vi "DerotatorControl_byYaw.vi"() -> ()   [LabVIEW 2020]
uses:
  <vilib>/DAQmx/write.llb/DAQmx Write (Digital Bool 1Line 1Point).vi
  <vilib>/DAQmx/create/channels.llb/DAQmx Create Channel (DO-Digital Output).vi
  <vilib>/DAQmx/miscellaneous.llb/DAQmx Fill In Error Info.vi
  GlobalYAW.vi
panel:
  in  "step":bool
  in  "stop":bool
  in  "Record!":bool
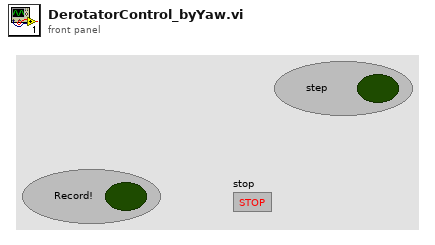
[diagram p1: front panel]
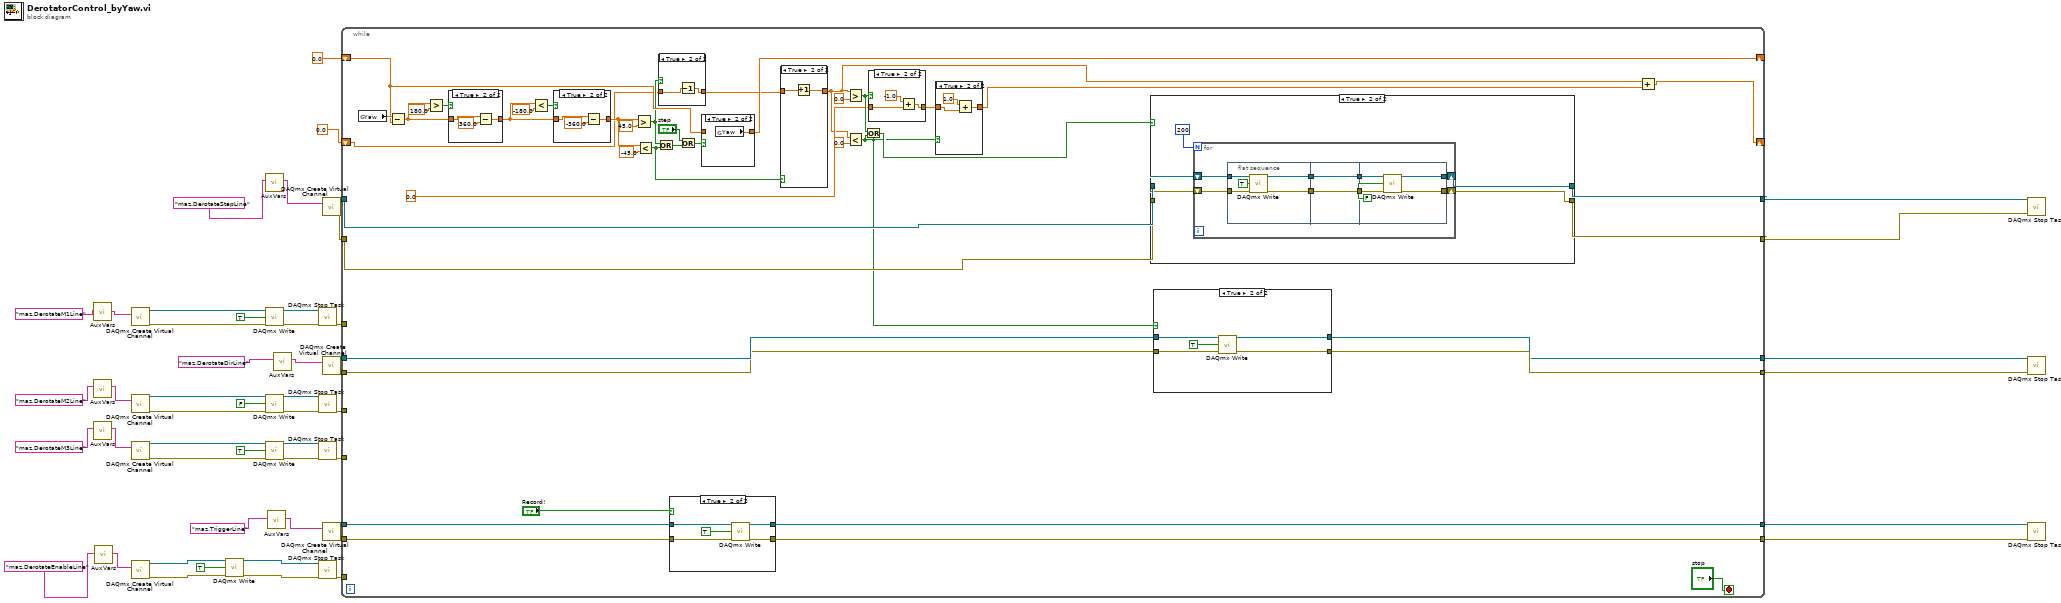
[diagram p0: block diagram]
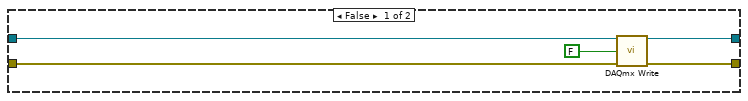
[diagram p9: hidden frame]
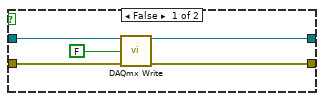
[diagram p10: hidden frame]
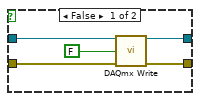
[diagram p11: hidden frame]
diagram:
  n1 = call "AuxVars.vi"("key"="maz.DerotateM1Line") -> ("value"=w15:string)  [unwired: 9 in, 1 out]
  n2 = call "AuxVars.vi"("key"="maz.DerotateM2Line") -> ("value"=w9:string)  [unwired: 9 in, 1 out]
  n3 = call "AuxVars.vi"("key"="maz.DerotateM3Line") -> ("value"=w7:string)  [unwired: 9 in, 1 out]
  n4 = call "AuxVars.vi"("key"="maz.DerotateEnableLine") -> ("value"=w5:string)  [unwired: 9 in, 1 out]
  n5 = call-poly <vilib>:"DAQmx Create Virtual Channel.vi"("lines"=w15) -> ("task out"=w34:refnum<k21>, "error out"=w31:errorcluster)  [unwired: 13 in]
  n6 = call-poly <vilib>:"DAQmx Create Virtual Channel.vi"("lines"=w9) -> ("task out"=w29:refnum<k21>, "error out"=w26:errorcluster)  [unwired: 13 in]
  n7 = call-poly <vilib>:"DAQmx Create Virtual Channel.vi"("lines"=w7) -> ("task out"=w24:refnum<k21>, "error out"=w21:errorcluster)  [unwired: 13 in]
  n8 = call-poly <vilib>:"DAQmx Create Virtual Channel.vi"("lines"=w5) -> ("task out"=w39:refnum<k21>, "error out"=w36:errorcluster)  [unwired: 13 in]
  n9 = call-poly <vilib>:"DAQmx Write.vi"("task/channels in"=w39, "data"=TRUE, "error in"=w36) -> ("task out"=w38:refnum<k21>, "error out"=w37:errorcluster)  [unwired: 10 in, 1 out]
  n10 = call "AuxVars.vi"("key"="maz.DerotateStepLine") -> ("value"=w13:string)  [unwired: 9 in, 1 out]
  n11 = call-poly <vilib>:"DAQmx Write.vi"("task/channels in"=w34, "data"=TRUE, "error in"=w31) -> ("task out"=w33:refnum<k21>, "error out"=w32:errorcluster)  [unwired: 10 in, 1 out]
  n12 = call-poly <vilib>:"DAQmx Write.vi"("task/channels in"=w29, "data"=FALSE, "error in"=w26) -> ("task out"=w28:refnum<k21>, "error out"=w27:errorcluster)  [unwired: 10 in, 1 out]
  n13 = call-poly <vilib>:"DAQmx Write.vi"("task/channels in"=w24, "data"=TRUE, "error in"=w21) -> ("task out"=w23:refnum<k21>, "error out"=w22:errorcluster)  [unwired: 10 in, 1 out]
  n14 = call "AuxVars.vi"("key"="maz.TriggerLine") -> ("value"=w3:string)  [unwired: 9 in, 1 out]
  n15 = call "AuxVars.vi"("key"="maz.DerotateDirLine") -> ("value"=w11:string)  [unwired: 9 in, 1 out]
  n16 = call <vilib>:"DAQmx Stop Task.vi"("task/channels in"=w33, "error in"=w32) -> ("error out"=w19:errorcluster)  [unwired: 12 in, 1 out]
  n17 = call <vilib>:"DAQmx Stop Task.vi"("task/channels in"=w28, "error in"=w27) -> ("error out"=w18:errorcluster)  [unwired: 12 in, 1 out]
  n18 = call <vilib>:"DAQmx Stop Task.vi"("task/channels in"=w23, "error in"=w22) -> ("error out"=w17:errorcluster)  [unwired: 12 in, 1 out]
  n19 = call <vilib>:"DAQmx Stop Task.vi"("task/channels in"=w38, "error in"=w37) -> ("error out"=w20:errorcluster)  [unwired: 12 in, 1 out]
  n20 = call-poly <vilib>:"DAQmx Create Virtual Channel.vi"("lines"=w13) -> ("task out"=w48:refnum<k21>, "error out"=w47:errorcluster)  [unwired: 13 in]
  n21 = call-poly <vilib>:"DAQmx Create Virtual Channel.vi"("lines"=w11) -> ("task out"=w44:refnum<k21>, "error out"=w43:errorcluster)  [unwired: 13 in]
  n22 = call-poly <vilib>:"DAQmx Create Virtual Channel.vi"("lines"=w3) -> ("task out"=w52:refnum<k21>, "error out"=w51:errorcluster)  [unwired: 13 in]
  n23 = while {
    tunnel: w52 -> [w95]
    tunnel: w51 -> [w94]
    tunnel: [w93] -> w50
    tunnel: [w92] -> w49
    tunnel: w48 -> [w90]
    tunnel: w47 -> [w89]
    tunnel: [w88] -> w46
    tunnel: [w87] -> w45
    tunnel: w44 -> [w86]
    tunnel: w43 -> [w85]
    tunnel: [w84] -> w42
    tunnel: [w83] -> w41
    tunnel: w20 -> [_]
    tunnel: w19 -> [_]
    tunnel: w18 -> [_]
    tunnel: w17 -> [_]
    shift-right: [w70] -> _
    shift-left: 0.0 ("Yaw") -> [w69]
    shift-right: [w54] -> _
    shift-left: 0.0 ("Yaw") -> [w61]
    stop <- "stop" stop-if-true
    n24 = global read "GlobalYAW.vi" "Yaw"() -> (w82:dbl)
    n25 = Subtract(x=w82, y=w69) -> (x-y=w76:dbl)
    n26 = Greater?(x=w76, y=180.0) -> (0:w75:bool)
    n27 = case shown="True" w75 {
      tunnel: w76 -> [w116 w119]
      tunnel: [w116 w117] -> w71
      frame False {
      }
      frame True {
        n28 = Subtract(x=w119, y=360.0) -> (x-y=w117:dbl)
      }
    }
    n29 = Less?(x=w71, y=-180.0) -> (x < y?=w72:bool)
    n30 = case shown="True" w72 {
      tunnel: w71 -> [w112 w115]
      tunnel: [w112 w113] -> w73
      frame False {
      }
      frame True {
        n31 = Subtract(x=w115, y=-360.0) -> (x-y=w113:dbl)
      }
    }
    n32 = Greater?(x=w73, y=45.0) -> (0:w63:bool)
    n33 = Less?(x=w73, y=-45.0) -> (x < y?=w62:bool)
    n34 = Or(x=w63, y=w62) -> (x .or. y?=w81:bool)
    n35 = case shown="True" w63 {
      tunnel: w61 -> [w104 w105]
      tunnel: [w104 w106] -> w68
      frame False {
      }
      frame True {
        n36 = Decrement(x=w105) -> (x-1=w106:dbl)
      }
    }
    n37 = case shown="True" "Record!" {
      tunnel: w95 -> [w163 w169]
      tunnel: w94 -> [w162 w168]
      tunnel: [w161 w167] -> w93
      tunnel: [w160 w166] -> w92
      frame False {
        n38 = call-poly <vilib>:"DAQmx Write.vi"("task/channels in"=w163, "data"=FALSE, "error in"=w162) -> ("task out"=w161:refnum<k21>, "error out"=w160:errorcluster)  [unwired: 10 in, 1 out]
      }
      frame True {
        n39 = call-poly <vilib>:"DAQmx Write.vi"("task/channels in"=w169, "data"=TRUE, "error in"=w168) -> ("task out"=w167:refnum<k21>, "error out"=w166:errorcluster)  [unwired: 10 in, 1 out]
      }
    }
    n40 = Or(x="step", y=w81) -> (x .or. y?=w65:bool)
    n41 = case shown="True" w65 {
      tunnel: [w110 w111] -> w70
      tunnel: w69 -> [w110 _]
      frame False {
      }
      frame True {
        n42 = global read "GlobalYAW.vi" "Yaw"() -> (w111:dbl)
      }
    }
    n43 = case shown="True" w62 {
      tunnel: w68 -> [w107 w108]
      tunnel: [w107 w109] -> w55
      frame False {
      }
      frame True {
        n44 = Increment(x=w108) -> (x+1=w109:dbl)
      }
    }
    n45 = Greater?(x=w55, y=0.0) -> (0:w59:bool)
    n46 = Less?(x=w55, y=0.0) -> (x < y?=w58:bool)
    n47 = Or(x=w59, y=w58) -> (x .or. y?=w64:bool)
    n48 = case shown="True" w59 {
      tunnel: 0.0 ("Yaw") -> [w100 w103]
      tunnel: [w100 w102] -> w60
      frame False {
      }
      frame True {
        n49 = Add(x=-1.0, y=w103) -> (x+y=w102:dbl)
      }
    }
    n50 = case shown="True" w58 {
      tunnel: w60 -> [w96 w99]
      tunnel: [w96 w98] -> w56
      frame False {
      }
      frame True {
        n51 = Add(x=1.0, y=w99) -> (x+y=w98:dbl)
      }
    }
    n52 = case shown="True" w64 {
      tunnel: w90 -> [w123 w129]
      tunnel: w89 -> [w122 w128]
      tunnel: [w121 w126] -> w87
      tunnel: [w120 w127] -> w88
      frame False {
        n53 = call-poly <vilib>:"DAQmx Write.vi"("task/channels in"=w123, "data"=FALSE, "error in"=w122) -> ("task out"=w121:refnum<k21>, "error out"=w120:errorcluster)  [unwired: 10 in, 1 out]
      }
      frame True {
        n54 = for {
          N: 200 -> [_]
          shift-right: [w130] -> w126
          shift-left: w129 -> [w133]
          shift-right: [w131] -> w127
          shift-left: w128 -> [w132]
          n55 = flat-sequence {
            tunnel: w133 -> [w141]
            tunnel: w132 -> [w140]
            tunnel: [w139] -> w137
            tunnel: [w138] -> w136
            tunnel: w137 -> [w144]
            tunnel: [w144] -> w135
            tunnel: w136 -> [w143]
            tunnel: [w143] -> w134
            tunnel: [w148] -> w130
            tunnel: [w146] -> w131
            tunnel: w135 -> [w147]
            tunnel: w134 -> [w149]
            frame #0 {
              n56 = call-poly <vilib>:"DAQmx Write.vi"("task/channels in"=w141, "data"=TRUE, "error in"=w140) -> ("task out"=w138:refnum<k21>, "error out"=w139:errorcluster)  [unwired: 10 in, 1 out]
            }
            frame #1 {
            }
            frame #2 {
              n57 = call-poly <vilib>:"DAQmx Write.vi"("task/channels in"=w149, "data"=FALSE, "error in"=w147) -> ("task out"=w148:refnum<k21>, "error out"=w146:errorcluster)  [unwired: 10 in, 1 out]
            }
          }
        }
      }
    }
    n58 = case shown="True" w58 {
      tunnel: w86 -> [w153 w159]
      tunnel: w85 -> [w152 w158]
      tunnel: [w151 w157] -> w83
      tunnel: [w150 w156] -> w84
      frame False {
        n59 = call-poly <vilib>:"DAQmx Write.vi"("task/channels in"=w153, "data"=FALSE, "error in"=w152) -> ("task out"=w151:refnum<k21>, "error out"=w150:errorcluster)  [unwired: 10 in, 1 out]
      }
      frame True {
        n60 = call-poly <vilib>:"DAQmx Write.vi"("task/channels in"=w159, "data"=TRUE, "error in"=w158) -> ("task out"=w157:refnum<k21>, "error out"=w156:errorcluster)  [unwired: 10 in, 1 out]
      }
    }
    n61 = Add(x=w55, y=w56) -> (x+y=w54:dbl)
  }
  n62 = call <vilib>:"DAQmx Stop Task.vi"("task/channels in"=w45, "error in"=w46) -> ()  [unwired: 12 in, 2 out]
  n63 = call <vilib>:"DAQmx Stop Task.vi"("task/channels in"=w41, "error in"=w42) -> ()  [unwired: 12 in, 2 out]
  n64 = call <vilib>:"DAQmx Stop Task.vi"("task/channels in"=w50, "error in"=w49) -> ()  [unwired: 12 in, 2 out]
